vi "switchQuene.vi"(0 "switchQuene In":refnum<queue>, 5 "switchIndexOffset":i32, 7 "pairStartIndex":i32, 9 "S-para Pair Name":string[](array[string]), 11 "错误输入（无错误）":errorcluster) -> (4 "switchQuene Out":refnum<queue>, 15 "error out":errorcluster)   [LabVIEW 2011]
uses:
  dataType/switchMsg.ctl
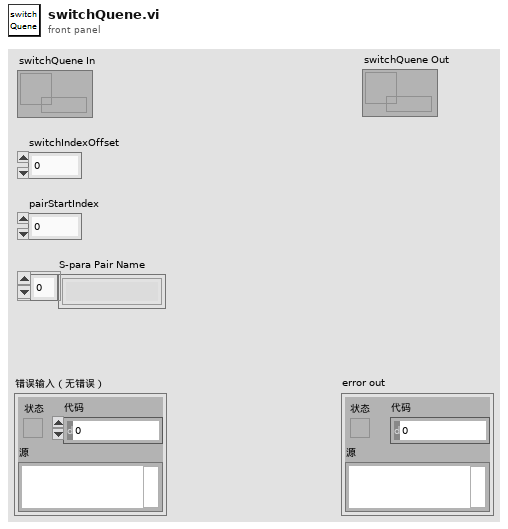
[diagram p1: front panel]
types:
  T1 = typedef "switchMsg.ctl" = cluster{"index":i32, "pairName":string, "switchIndex":i32, "TestAction":enum16{"start", "stop", "pause", "reset"}}
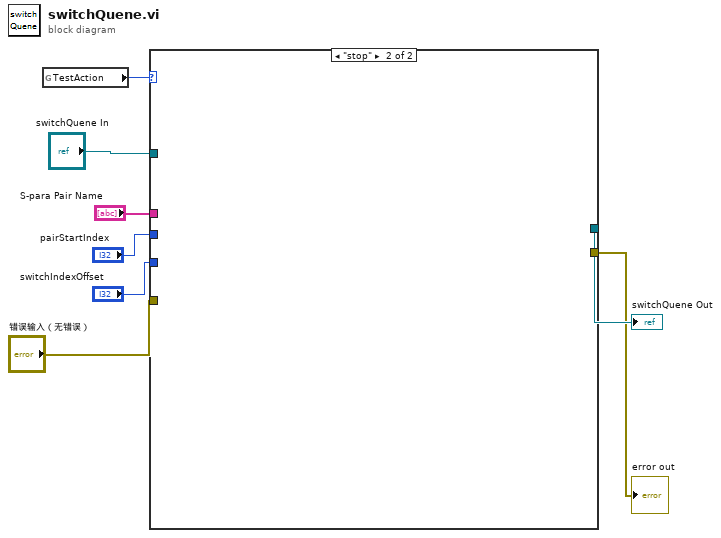
[diagram p0: block diagram]
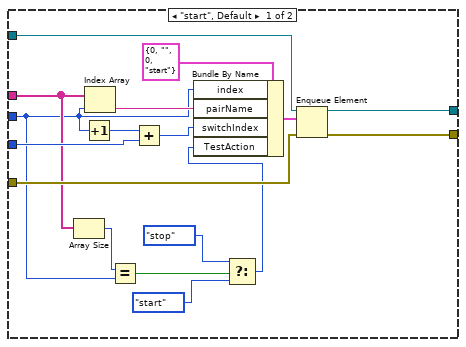
[diagram p2: hidden frame]
diagram:
  n1 = global read "全局.vi" "TestAction"() -> (w4:enum16{"start", "stop", "pause", "reset"})
  n2 = case shown="\"stop\"" w4 {
    tunnel: "switchQuene In" -> [w19 _]
    tunnel: "S-para Pair Name" -> [w15 _]
    tunnel: "pairStartIndex" -> [w13 _]
    tunnel: "switchIndexOffset" -> [w21 _]
    tunnel: [w18 _] -> w8
    tunnel: "错误输入（无错误）" -> [w17 _]
    tunnel: [w16 _] -> w1
    frame "start", Default {
      n3 = Array Size(array=w15) -> (size(s)=w14:i32)
      n4 = Increment(x=w13) -> (x+1=w22:i32)
      n5 = Index Array(array=w15, index=w13) -> (element=w23:string)
      n6 = Equal?(x=w14, y=w13) -> (x = y?=w12:bool)
      n7 = Add(x=w22, y=w21) -> (x+y=w20:i32)
      n8 = Select(t=enum16{"start", "stop", "pause", "reset"}."stop" ("TestAction"), s=w12, f=enum16{"start", "stop", "pause", "reset"}."start" ("TestAction")) -> (s? t:f=w9:enum16{"start", "stop", "pause", "reset"})
      n9 = Bundle By Name(cluster=T1 {"index"=0, "pairName"="", "switchIndex"=0, "TestAction"=enum."start"} ("switchMsg"), "index"=w13, "pairName"=w23, "switchIndex"=w20, "TestAction"=w9) -> (w24:T1)
      n10 = Enqueue Element(queue=w19, element=w24, error in (no error)=w17) -> (queue out=w18:refnum<queue>, error out=w16:errorcluster)  [unwired: 1 in, 1 out]
    }
    frame "stop" {
    }
  }
  "switchQuene Out" <- w8
  "error out" <- w1
